vi "BoltekInStr.vi"(2 "Offset":dbl format="%.1f", 3 "read buffer":string, 4 "controllo_segno":bool) -> (0 "kV/m":string, 1 "mV":string)   [LabVIEW 2010]
panel:
  out "tampone":string
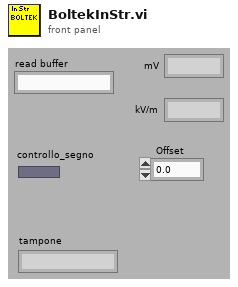
[diagram p1: front panel]
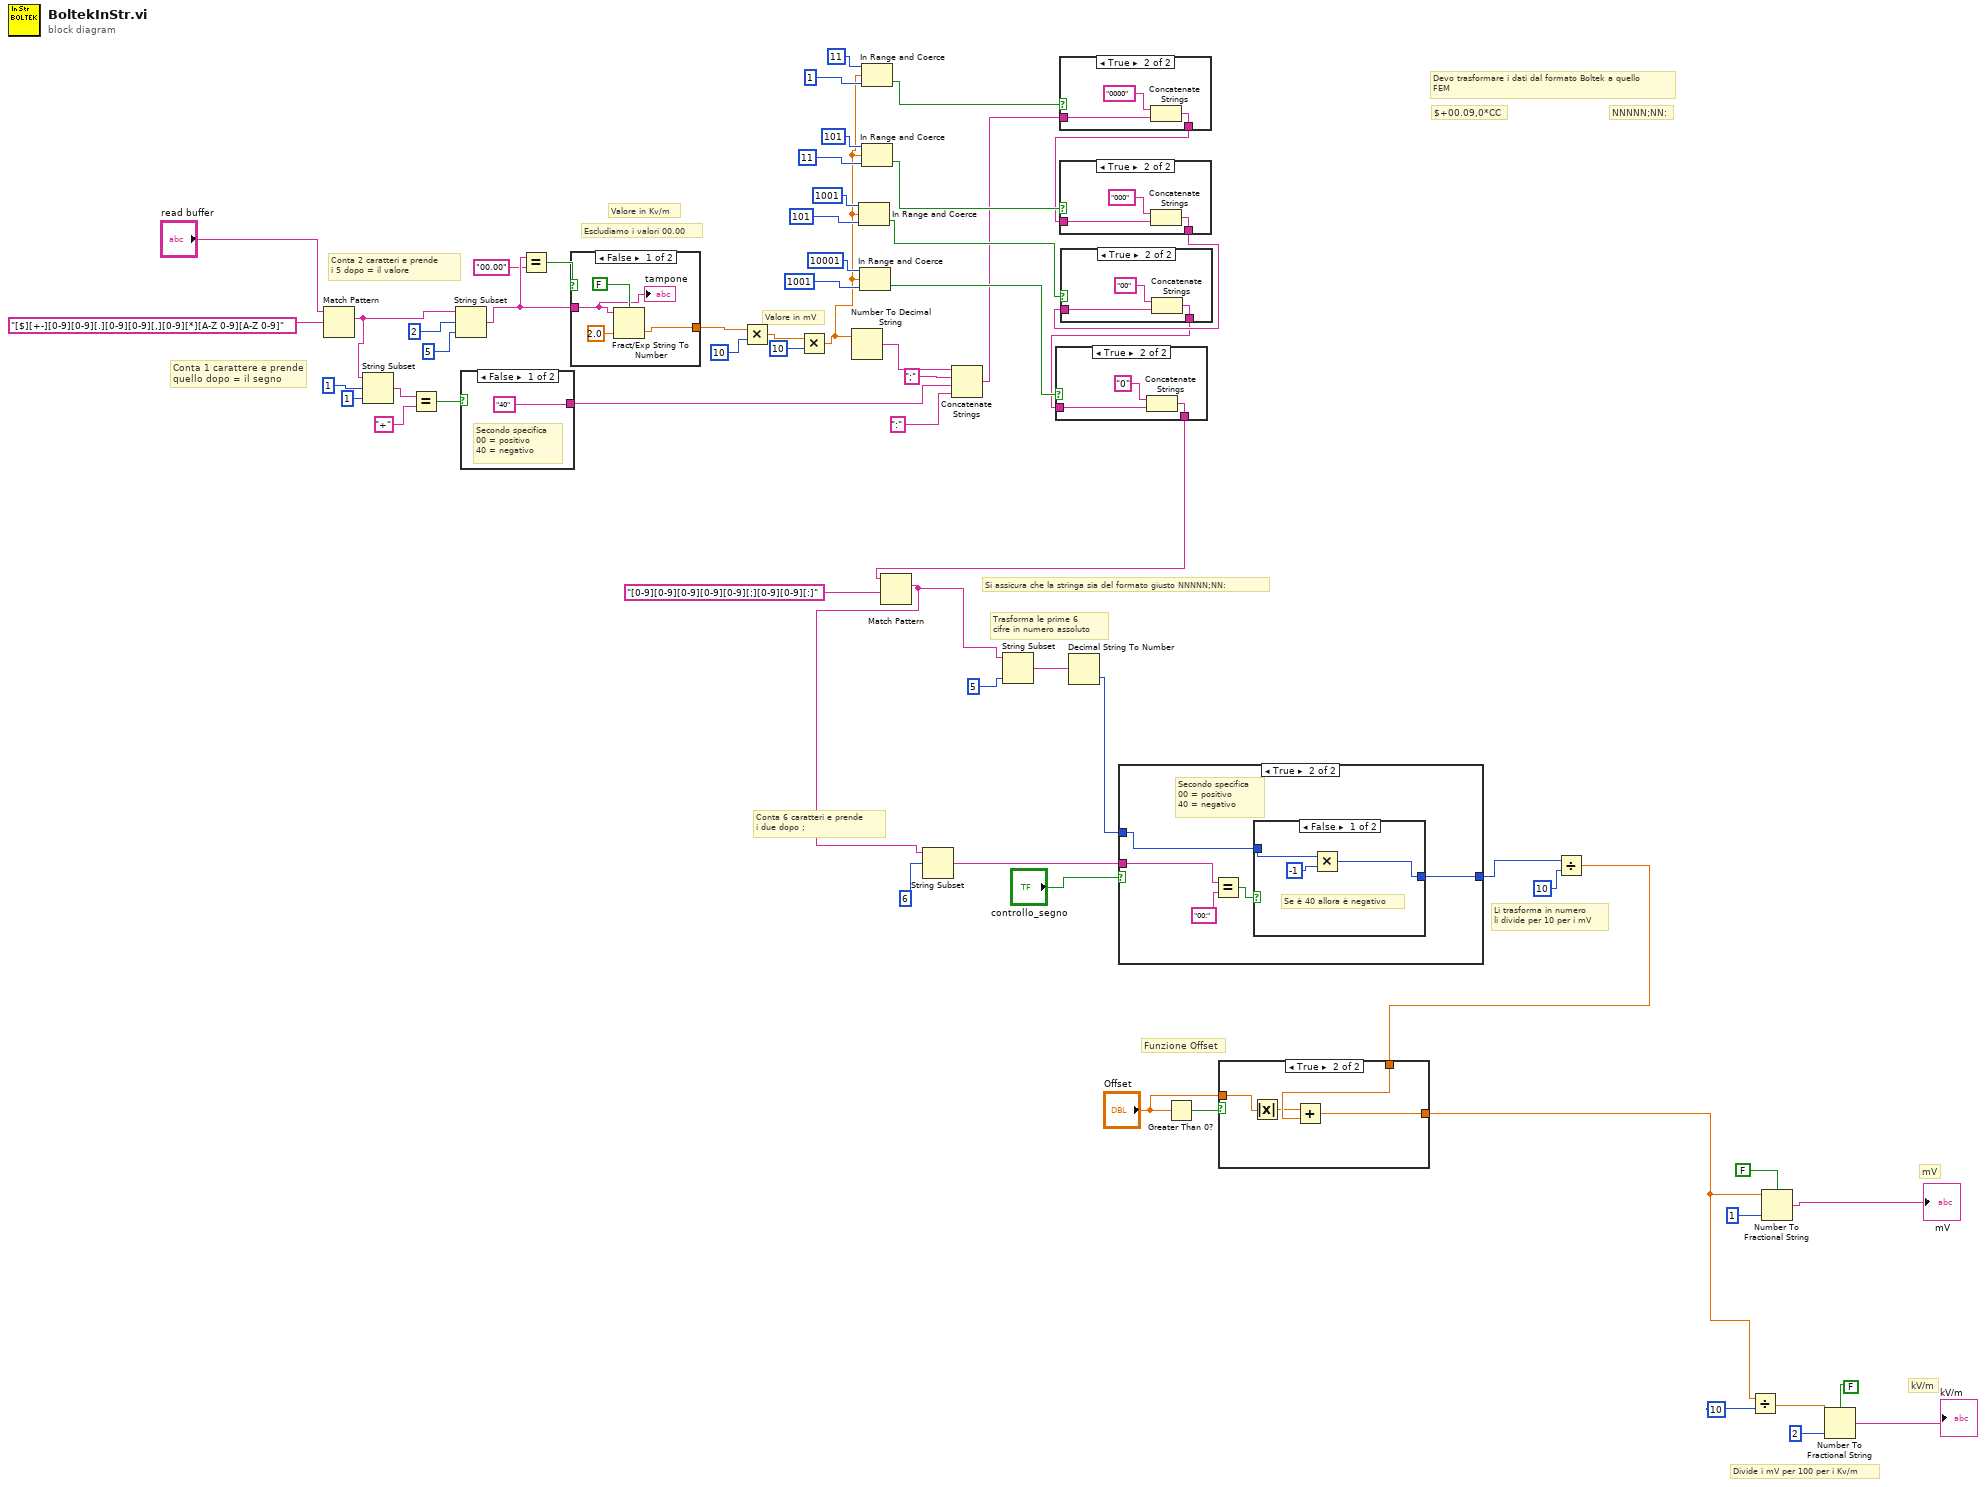
[diagram p0: block diagram]
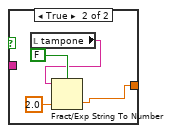
[diagram p2: hidden frame]
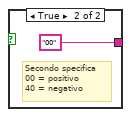
[diagram p7: hidden frame]
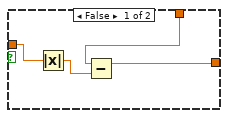
[diagram p8: hidden frame]
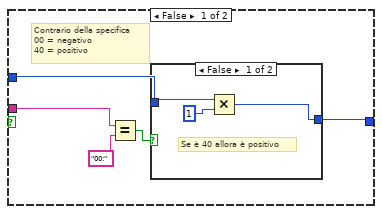
[diagram p9: hidden frame]
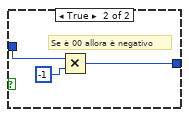
[diagram p10: hidden frame]
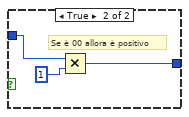
[diagram p11: hidden frame]
diagram:
  # "Escludiamo i valori 00.00"
  # "Valore in Kv/m"
  # "Valore in mV"
  # "Conta 2 caratteri e prende\ni 5 dopo = il valore"
  # "Conta 1 carattere e prende\nquello dopo = il segno"
  # "NNNNN;NN:"
  # "Devo trasformare i dati dal formato Boltek a quello\nFEM"
  # "$+00.09,0*CC"
  # "kV/m"
  # "mV"
  # "Funzione Offset"
  # "Li trasforma in numero\nli divide per 10 per i mV"
  # "Trasforma le prime 6\ncifre in numero assoluto"
  # "Divide i mV per 100 per i Kv/m"
  # "Conta 6 caratteri e prende\ni due dopo ;"
  # "Si assicura che la stringa sia del formato giusto NNNNN;NN:"
  n1 = Match Pattern(string="read buffer", regular expression="[$][+-][0-9][0-9][.][0-9][0-9][,][0-9][*][A-Z 0-9][A-Z 0-9]") -> (match substring=w33:string)  [unwired: 1 in, 3 out]
  n2 = String Subset(string=w33, offset (0)=1, length (rest)=1 ("length (rest)")) -> (substring=w36:string)
  n3 = Equal?(x=w36, y="+") -> (x = y?=w34:bool)
  n4 = String Subset(string=w33, offset (0)=2, length (rest)=5) -> (substring=w2:string)
  n5 = case shown="False" w34 {
    tunnel: ["40" "00"] -> w25
    frame False {
      # "Secondo specifica\n00 = positivo\n40 = negativo"
    }
    frame True {
      # "Secondo specifica\n00 = positivo\n40 = negativo"
    }
  }
  n6 = Equal?(x=w2, y="00.00") -> (x = y?=w3:bool)
  n7 = case shown="False" w3 {
    tunnel: w2 -> [w64 _]
    tunnel: [w65 w68] -> w4
    frame False {
      n8 = Fract/Exp String To Number(use system decimal point (T)=FALSE, string=w64, default (0 dbl)=2.0 ("default (0 DBL)")) -> (number=w65:dbl)  [unwired: 1 in, 1 out]
      "tampone" <- w64
    }
    frame True {
      n9 = local read "tampone"() -> (w69:string)
      n10 = Fract/Exp String To Number(use system decimal point (T)=FALSE, string=w69, default (0 dbl)=2.0 ("default (0 DBL)")) -> (number=w68:dbl)  [unwired: 1 in, 1 out]
    }
  }
  n11 = Multiply(x=w4, y=10) -> (x*y=w29:dbl)
  n12 = Multiply(x=w29, y=10) -> (x*y=w13:dbl)
  n13 = Number To Decimal String(number=w13) -> (decimal integer string=w27:string)  [unwired: 1 in]
  n14 = In Range and Coerce(upper limit=1001, x=w13, lower limit=101) -> (In Range?=w11:bool)  [unwired: 1 out]
  n15 = In Range and Coerce(upper limit=10001, x=w13, lower limit=1001) -> (In Range?=w21:bool)  [unwired: 1 out]
  n16 = In Range and Coerce(upper limit=11, x=w13, lower limit=1) -> (In Range?=w12:bool)  [unwired: 1 out]
  n17 = In Range and Coerce(upper limit=101, x=w13, lower limit=11) -> (In Range?=w10:bool)  [unwired: 1 out]
  n18 = Concatenate Strings(w27, ";" ("string"), w25, ":" ("string")) -> (w9:string)
  n19 = case shown="True" w12 {
    tunnel: w9 -> [w72 w74]
    tunnel: [w72 w73] -> w8
    frame False {
    }
    frame True {
      n20 = Concatenate Strings("0000" ("string"), w74) -> (w73:string)
    }
  }
  n21 = case shown="True" w10 {
    tunnel: w8 -> [w76 w78]
    tunnel: [w76 w77] -> w7
    frame False {
    }
    frame True {
      n22 = Concatenate Strings("000" ("string"), w78) -> (w77:string)
    }
  }
  n23 = case shown="True" w11 {
    tunnel: w7 -> [w80 w82]
    tunnel: [w80 w81] -> w6
    frame False {
    }
    frame True {
      n24 = Concatenate Strings("00" ("string"), w82) -> (w81:string)
    }
  }
  n25 = case shown="True" w21 {
    tunnel: w6 -> [w84 w86]
    tunnel: [w84 w85] -> w20
    frame False {
    }
    frame True {
      n26 = Concatenate Strings("0" ("string"), w86) -> (w85:string)
    }
  }
  n27 = Match Pattern(string=w20, regular expression="[0-9][0-9][0-9][0-9][0-9][;][0-9][0-9][:]" ("format string")) -> (match substring=w49:string)  [unwired: 1 in, 3 out]
  n28 = String Subset(string=w49, offset (0)=6) -> (substring=w47:string)  [unwired: 1 in]
  n29 = String Subset(string=w49, length (rest)=5) -> (substring=w54:string)  [unwired: 1 in]
  n30 = Decimal String To Number(string=w54) -> (number=w46:i32)  [unwired: 2 in, 1 out]
  n31 = case shown="True" "controllo_segno" {
    tunnel: w47 -> [w90 w102]
    tunnel: w46 -> [w89 w99]
    tunnel: [w88 w100] -> w45
    frame False {
      # "Contrario della specifica\n00 = negativo\n40 = positivo"
      n32 = Equal?(x=w90, y="00:") -> (x = y?=w91:bool)
      n33 = case shown="False" w91 {
        tunnel: w89 -> [w94 w97]
        tunnel: [w93 w96] -> w88
        frame False {
          # "Se è 40 allora è positivo"
          n34 = Multiply(x=w94, y=1) -> (x*y=w93:i32)
        }
        frame True {
          # "Se è 00 allora è negativo"
          n35 = Multiply(x=w97, y=-1) -> (x*y=w96:i32)
        }
      }
    }
    frame True {
      # "Secondo specifica\n00 = positivo\n40 = negativo"
      n36 = Equal?(x=w102, y="00:") -> (x = y?=w101:bool)
      n37 = case shown="False" w101 {
        tunnel: w99 -> [w105 w107]
        tunnel: [w104 w108] -> w100
        frame False {
          # "Se è 40 allora è negativo"
          n38 = Multiply(x=w105, y=-1) -> (x*y=w104:i32)
        }
        frame True {
          # "Se è 00 allora è positivo"
          n39 = Multiply(x=w107, y=1) -> (x*y=w108:i32)
        }
      }
    }
  }
  n40 = Greater Than 0?(x="Offset") -> (x > 0?=w43:bool)
  n41 = Divide(x=w45, y=10) -> (x/y=w41:dbl)
  n42 = case shown="True" w43 {
    tunnel: "Offset" -> [w110 w117]
    tunnel: w41 -> [w113 w116]
    tunnel: [w111 w114] -> w40
    frame False {
      n43 = Absolute Value(x=w110) -> (abs(x)=w112:dbl)
      n44 = Subtract(x=w113, y=w112) -> (x-y=w111:dbl)
    }
    frame True {
      n45 = Absolute Value(x=w117) -> (abs(x)=w115:dbl)
      n46 = Add(x=w115, y=w116) -> (x+y=w114:dbl)
    }
  }
  n47 = Divide(x=w40, y=10) -> (x/y=w59:dbl)
  n48 = Number To Fractional String(use system decimal point (T)=FALSE, number=w40, precision (6)=1) -> (F-format string=→"mV":string)  [unwired: 1 in]
  n49 = Number To Fractional String(use system decimal point (T)=FALSE, number=w59, precision (6)=2) -> (F-format string=→"kV/m":string)  [unwired: 1 in]
